vi "Configure Trigger.vi"() -> ()   [LabVIEW 2023, in "HAL.lvlib" / "Scope PXI.lvlib" / "Scope PXI CFG.lvclass"]
uses:
  Scope PXI CFG.lvclass
  Scope PXI CFG.lvclass/Scope PXI CFG.ctl
  Configuration Base/Configuration Base.lvclass
  <vilib>/Utility/error.llb/Error Cluster From Error Code.vi
  <vilib>/ErrorRing/Error Ring.xnode
  4b4b6126-2405-414b-91da-33c74864ffaf.vi
  d6385bd9-32f1-4e86-8d66-f1f6b280b9ec.vi
  795efc06-cdc5-4534-8f89-f6f4812d0b8b.vi
  <vilib>/JDP Science/JSONtext/JSONtext.lvlib
  <instrlib>/niScope/Configure/Trigger/niScope Configure Trigger Digital.vi
  <instrlib>/niScope/Controls/niScope trigger source digital.ctl
  733de5b7-6890-4c28-a56b-02f88581e263.vi
  <instrlib>/niScope/Configure/Trigger/niScope Configure Trigger Software.vi
  765cffe9-2255-4ad2-9e07-50fe9ea097c6.vi
  <instrlib>/niScope/Controls/niScope trigger slope.ctl
  D:/git/HAL/Configuration Base/Configuration Base.lvclass
  D:/git/HAL/Interfaces/IConfigure/IConfigure.lvclass
  D:/git/HAL/Scope PXI/Scope PXI CFG/Scope PXI CFG.lvclass
panel:
  out "Scope PXI CFG out":refnum<class "Scope PXI CFG.lvclass">
  in  "Scope PXI CFG in":refnum<class "Scope PXI CFG.lvclass">
  out "error out":errorcluster
  in  "error in":errorcluster
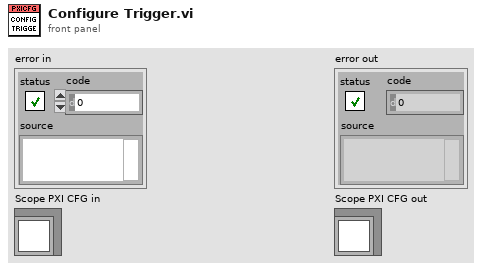
[diagram p1: front panel]
types:
  T1 = typedef "niScope trigger slope.ctl" = i32
  T2 = typedef "niScope trigger source digital.ctl" = string
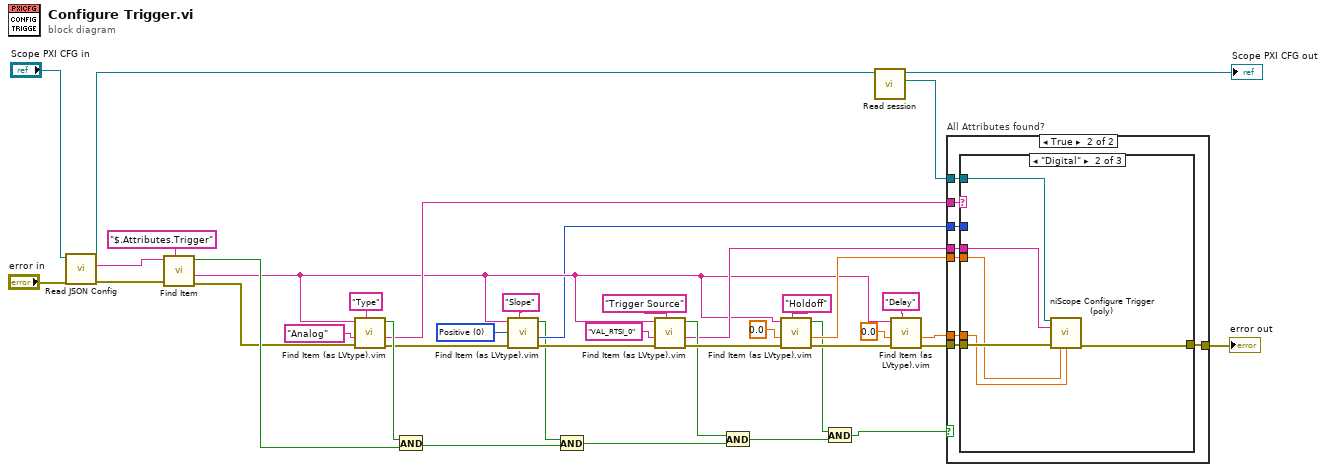
[diagram p0: block diagram]
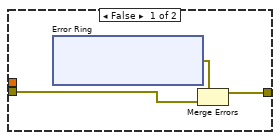
[diagram p2: hidden frame]
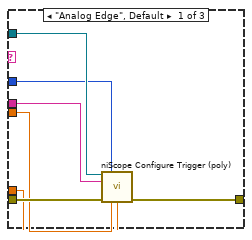
[diagram p3: hidden frame]
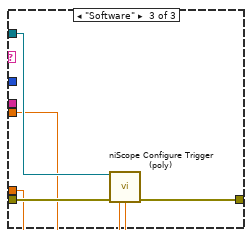
[diagram p4: hidden frame]
diagram:
  w6 = T1 0 items=["Positive", "Negative"] ("trigger slope")
  n1 = call "Read JSON Config.vi"("error in"="error in", "object in"="Scope PXI CFG in") -> ("error out"=w39:errorcluster, "<JSON>Config"=w36:string, "object out"=w37:refnum<class "Scope PXI CFG.lvclass">)  [unwired: 7 in]
  n2 = call <vilib>:"Find Item.vi"("$Path or Item Name"="$.Attributes.Trigger", "error in (no error)"=w39, "JSON"=w36) -> ("error out"=w34:errorcluster, "<JSON>"=w5:string, "Found"=w35:bool)  [unwired: 5 in, 1 out]
  n3 = call "Find Item (as LVtype).vim"("$Path or Item Name"="Type", "error in (no error)"=w34, "Data Type and Default Value"="Analog" ("Type"), "JSON"=w5) -> ("error out"=w8:errorcluster, "Data"=w16:string, "Found"=w27:bool)  [unwired: 4 in, 1 out]
  n4 = And(x=w27, y=w35) -> (x .and. y?=w25:bool)
  n5 = call "Find Item (as LVtype).vim"("$Path or Item Name"="Slope", "error in (no error)"=w8, "Data Type and Default Value"=w6, "JSON"=w5) -> ("error out"=w7:errorcluster, "Data"=w4:T1, "Found"=w2:bool)  [unwired: 4 in, 1 out]
  n6 = And(x=w2, y=w25) -> (x .and. y?=w3:bool)
  n7 = call "Find Item (as LVtype).vim"("$Path or Item Name"="Trigger Source", "error in (no error)"=w7, "Data Type and Default Value"=T2 "VAL_RTSI_0" ("trigger source"), "JSON"=w5) -> ("error out"=w30:errorcluster, "Data"=w15:T2, "Found"=w26:bool)  [unwired: 4 in, 1 out]
  n8 = And(x=w26, y=w3) -> (x .and. y?=w23:bool)
  n9 = call "Find Item (as LVtype).vim"("$Path or Item Name"="Holdoff", "error in (no error)"=w30, "Data Type and Default Value"=0.0, "JSON"=w5) -> ("error out"=w29:errorcluster, "Data"=w28:dbl, "Found"=w24:bool)  [unwired: 4 in, 1 out]
  n10 = And(x=w24, y=w23) -> (x .and. y?=w18:bool)
  n11 = call "Read session.vi"("Scope PXI CFG in"=w37) -> ("session"=w38:refnum<k15>, "Scope PXI CFG out"=→"Scope PXI CFG out":refnum<class "Scope PXI CFG.lvclass">)  [unwired: 8 in, 1 out]
  n12 = call "Find Item (as LVtype).vim"("$Path or Item Name"="Delay", "error in (no error)"=w29, "Data Type and Default Value"=0.0, "JSON"=w5) -> ("error out"=w12:errorcluster, "Data"=w11:dbl)  [unwired: 4 in, 2 out]
  n13 = case "All Attributes found?" shown="True" w18 {
    tunnel: w12 -> [w41 w55]
    tunnel: w15 -> [_ w53]
    tunnel: [w42 w54] -> w20
    tunnel: w28 -> [_ w52]
    tunnel: w38 -> [_ w56]
    tunnel: w16 -> [_ w51]
    tunnel: w11 -> [_ w50]
    tunnel: w4 -> [_ w49]
    frame False {
      n14 = xnode "Error Ring"() -> ("error out"=w43:errorcluster)
      n15 = Merge Errors(w43, w41) -> (w42:errorcluster)
    }
    frame True {
      n16 = case shown="\"Digital\"" w51 {
        tunnel: w56 -> [w61 w66 w74]
        tunnel: w55 -> [w63 w69 w73]
        tunnel: [w62 w68 w72] -> w54
        tunnel: w53 -> [w60 w67 _]
        tunnel: w52 -> [w58 w65 w71]
        tunnel: w50 -> [w59 w64 w70]
        tunnel: w49 -> [w57 _ _]
        frame "Analog Edge", Default {
          n17 = call-poly <instrlib>:"niScope Configure Trigger (poly).vi"("instrument handle"=w61, "trigger slope"=w57, "trigger source"=w60, "error in"=w63, "trigger holdoff"=w58, "trigger delay"=w59) -> ("error out"=w62:errorcluster)  [unwired: 8 in, 1 out]
        }
        frame "Digital" {
          n18 = call-poly <instrlib>:"niScope Configure Trigger (poly).vi"("instrument handle"=w66, "trigger source"=w67, "error in"=w69, "trigger holdoff"=w65, "trigger delay"=w64) -> ("error out"=w68:errorcluster)  [unwired: 9 in, 1 out]
        }
        frame "Software" {
          n19 = call-poly <instrlib>:"niScope Configure Trigger (poly).vi"("instrument handle"=w74, "error in"=w73, "trigger holdoff"=w71, "trigger delay"=w70) -> ("error out"=w72:errorcluster)  [unwired: 10 in, 1 out]
        }
      }
    }
  }
  "error out" <- w20
